vi "DAQInit.vi"(3 "error in":errorcluster caption="entrée d'erreur", 5 "configInput":T1) -> (0 "error out":errorcluster caption="sortie d'erreur", 2 "task out":refnum<k21> caption="tâche en sortie")   [LabVIEW 2017]
uses:
  DefDeType/ConfigTotale.ctl
  DefDeType/VoltageChannels.ctl
  DefDeType/WBridgeChannels.ctl
  DefDeType/Configuration.ctl
  <vilib>/DAQmx/create/scale.llb/DAQmx Create Scale (Linear).vi
  <vilib>/DAQmx/create/channels.llb/DAQmx Create Channel (AI-Voltage-Basic).vi
  <vilib>/DAQmx/configure/timing.llb/DAQmx Timing (Sample Clock).vi
panel:
  out "nbVoies":i32
  out "Freq éch":u32
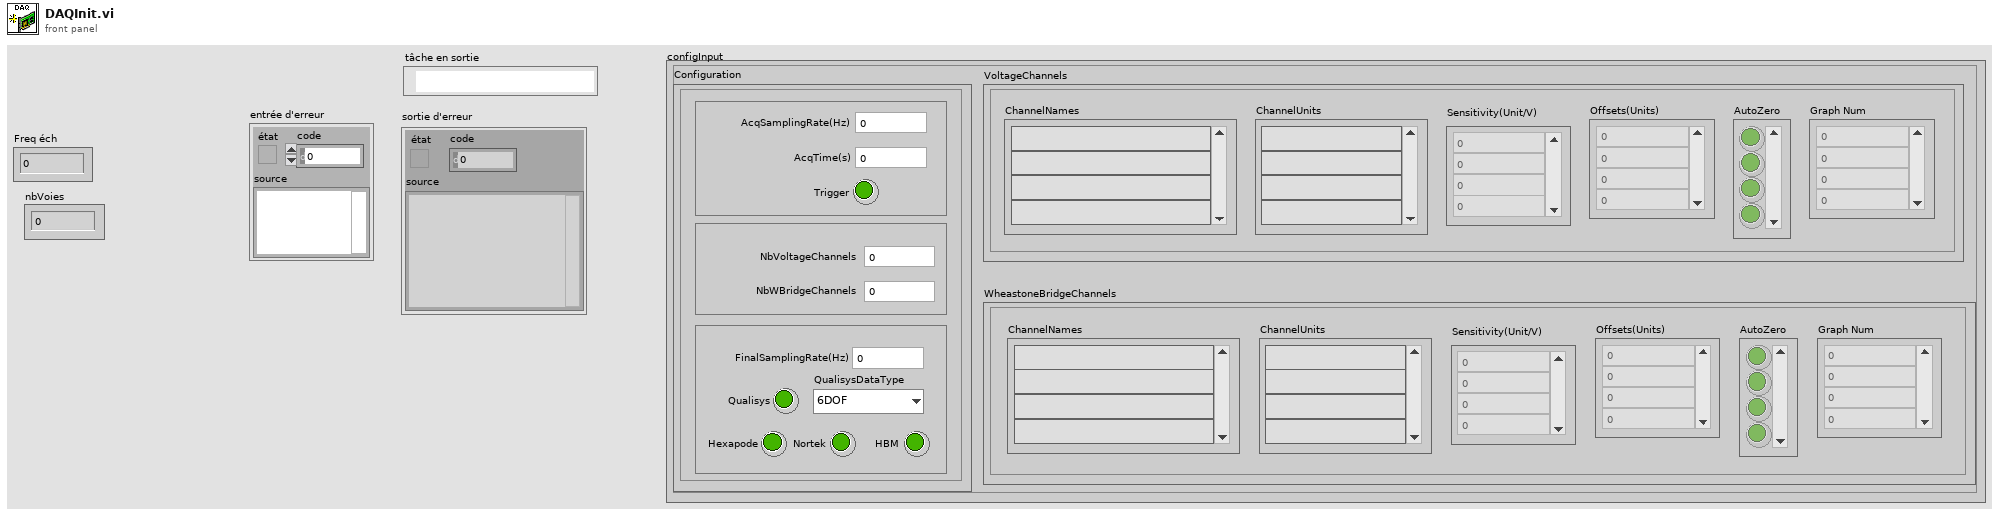
[diagram p1: front panel]
types:
  T1 = typedef "ConfigTotale.ctl" = cluster{"VoltageChannels":T2, "WheastoneBridgeChannels":T3, "Configuration":T4}
  T2 = typedef "VoltageChannels.ctl" = cluster{"ChannelNames":string[], "Sensitivity(Unit/V)":dbl[], "AutoZero":bool[], "ChannelUnits":string[], "Offsets(Units)":dbl[], "Graph Num":u8[]}
  T3 = typedef "WBridgeChannels.ctl" = cluster{"ChannelNames":string[], "Sensitivity(Unit/V)":dbl[], "AutoZero":bool[], "ChannelUnits":string[], "Offsets(Units)":dbl[], "Graph Num":u8[]}
  T4 = typedef "Configuration.ctl" = cluster{"AcqSamplingRate(Hz)":u32, "AcqTime(s)":u32, "Trigger":bool, "NbVoltageChannels":u32, "NbWBridgeChannels":u32, "Qualisys":bool, "Hexapode":bool, "FinalSamplingRate(Hz)":u32, "QualisysDataType":enum16{"6DOF", "3DTracking", "6DOF + 3D"}, "Nortek":bool, "HBM":bool}
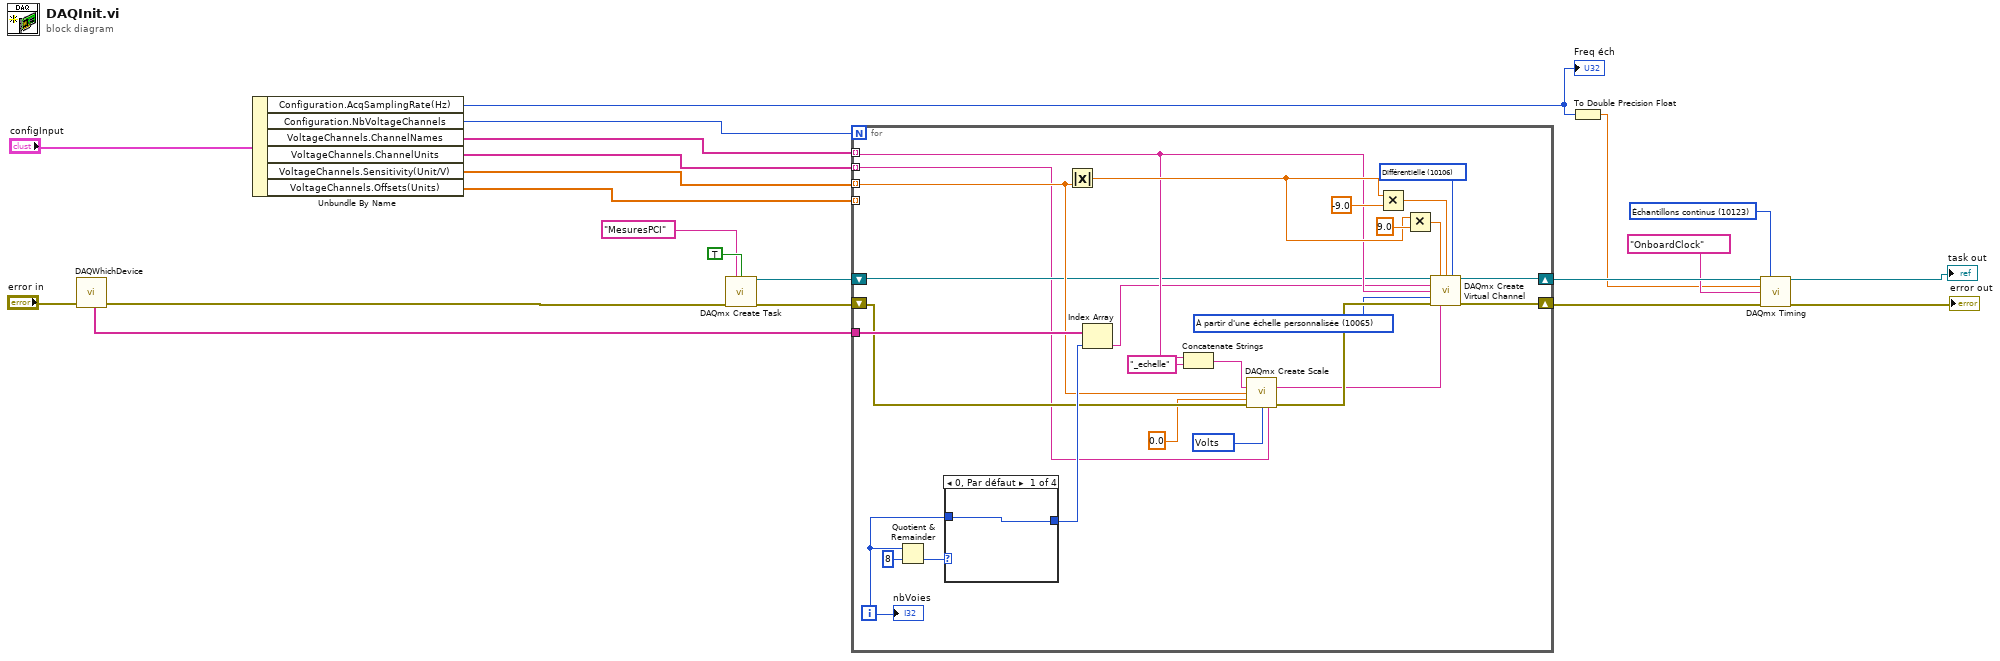
[diagram p0: block diagram]
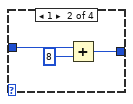
[diagram p2: hidden frame]
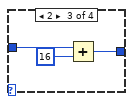
[diagram p3: hidden frame]
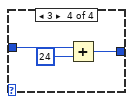
[diagram p4: hidden frame]
diagram:
  w17 = 10123 items=["Échantillons finis"=10178, "Échantillons continus"=10123, "Point par point avec cadencement matériel"=12522] ("sample mode")
  n1 = call "DAQWhichDevice.vi"("error in"="error in") -> ("error out"=w1:errorcluster, "AI.VoiesPhysiques"=w14:tag[])  [unwired: 1 in, 5 out]
  n2 = Unbundle By Name("configInput") -> ("Configuration.AcqSamplingRate(Hz)"=w8:u32, "Configuration.NbVoltageChannels"=w7:u32, "VoltageChannels.ChannelNames"=w6:string[], "VoltageChannels.ChannelUnits"=w5:string[], "VoltageChannels.Sensitivity(Unit/V)"=w4:dbl[], "VoltageChannels.Offsets(Units)"=w3:dbl[])
  "Freq éch" <- w8
  n3 = call <vilib>:"DAQmx Create Task.vi"("new task name"="MesuresPCI", "auto cleanup"=TRUE, "error in"=w1) -> ("task out"=w20:refnum<k21>, "error out"=w21:errorcluster)  [unwired: 11 in]
  n4 = for {
    N: w7 -> [_]
    shift-right: [w26] -> w18
    shift-left: w21 -> [w28]
    shift-right: [w27] -> w19
    shift-left: w20 -> [w25]
    tunnel: w14 -> [w44]
    tunnel: w6 -> [w30] mode=indexing
    tunnel: w5 -> [w23] mode=indexing
    tunnel: w4 -> [w29] mode=indexing
    tunnel: w3 -> [_] mode=indexing
    i -> [w45]
    w36 = 10065 items=["Volts"=10348, "À partir d'une échelle personnalisée"=10065] ("units")
    w37 = 10348 items=["Volts"=10348, "Amps"=10342, "Deg F"=10144, "Deg C"=10143, "Deg R"=10145, "Kelvins"=10325, "Déformation"=10299, "Ohms"=10384, "Hz"=10373, "Secondes"=10364, "Mètres"=10219, "Pouces"=10379, "Degrés"=10146, "Radians"=10273, "Tops"=10304, "g"=10186, "m/s^2"=12470, "Pascals"=10081, "Newtons"=15875, "Livres"=15876, "kgf"=15877, "psi"=15879, "bar"=15880, "Nm"=15881, "oz-po"=15882, "lb-po"=15883, "lb-ft"=15884, "Volts/Volt"=15896, "mVolts/Volt"=15897, "À partir de TEDS"=12516] ("pre-scaled units")
    w42 = 10106 items=["défaut"=-1, "RSE"=10083, "NRSE"=10078, "Différentielle"=10106, "Pseudodifférentielle"=12529] ("input terminal configuration")
    n5 = Quotient & Remainder(x=w45, y=8) -> (floor(x/y)=w46:i32)  [unwired: 1 out]
    n6 = case shown="0, Par défaut" w46 {
      tunnel: [w48 w50 w53 w56] -> w43
      tunnel: w45 -> [w48 w51 w54 w57]
      frame 0, Default {
      }
      frame 1 {
        n7 = Add(x=w51, y=8) -> (x+y=w50:i32)
      }
      frame 2 {
        n8 = Add(x=w54, y=16) -> (x+y=w53:i32)
      }
      frame 3 {
        n9 = Add(x=w57, y=24) -> (x+y=w56:i32)
      }
    }
    n10 = Absolute Value(x=w29) -> (abs(x)=w31:dbl)
    n11 = Index Array(array=w44, index=w43) -> (element=w24:tag)
    n12 = Concatenate Strings(w30, "_echelle" ("chaîne")) -> (w40:string)
    n13 = call-poly <vilib>:"DAQmx Create Scale.vi"("name"=w40, "slope"=w29, "y-intercept"=0.0, "error in"=w28, "pre-scaled units"=w37, "scaled units"=w23) -> ("scale out"=w38:tag, "error out"=w39:errorcluster)  [unwired: 8 in]
    n14 = Multiply(x=w31, y=-9.0) -> (x*y=w33:dbl)
    n15 = Multiply(x=w31, y=9.0) -> (x*y=w32:dbl)
    n16 = call-poly <vilib>:"DAQmx Create Virtual Channel.vi"("task in"=w25, "maximum value"=w32, "minimum value"=w33, "input terminal configuration"=w42, "physical channels"=w24, "name to assign"=w30, "units"=w36, "error in"=w39, "custom scale name"=w38) -> ("task out"=w27:refnum<k21>, "error out"=w26:errorcluster)  [unwired: 5 in]
    "nbVoies" <- w45
  }
  n17 = To Double Precision Float(number=w8) -> (double precision float=w13:dbl)
  n18 = call-poly <vilib>:"DAQmx Timing.vi"("task/channels in"=w19, "sample mode"=w17, "rate"=w13, "source"=tag "OnboardClock", "error in"=w18) -> ("task out"=→"task out":refnum<k21>, "error out"=→"error out":errorcluster)  [unwired: 9 in]
